vi "ErrorHandling.sendErrorEventToUI.vi"(0 "ErrorHandling in":refnum<class "ErrorHandling.lvclass">, 5 "error in (no error)":errorcluster) -> (14 "ErrorHandling out":refnum<class "ErrorHandling.lvclass">, 19 "error out":errorcluster)   [LabVIEW 2016, in "ErrorHandling.lvclass"]
doc: "Sendet das Ereignis \"errorOccurred\" an das optionale UI ErrorUI\n\n15.04.14 / sige"
uses:
  ErrorHandling.lvclass
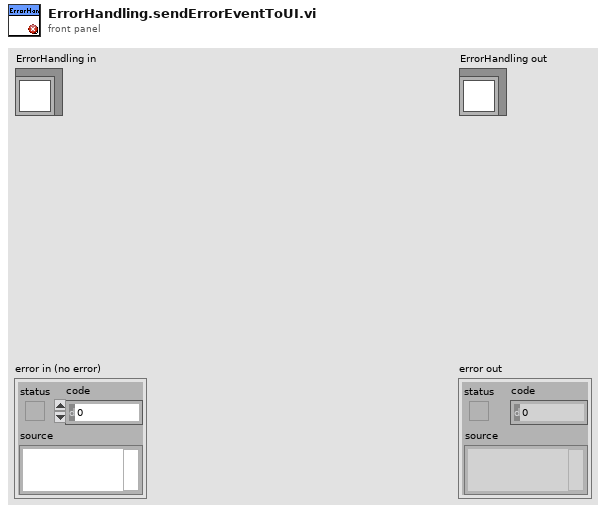
[diagram p1: front panel]
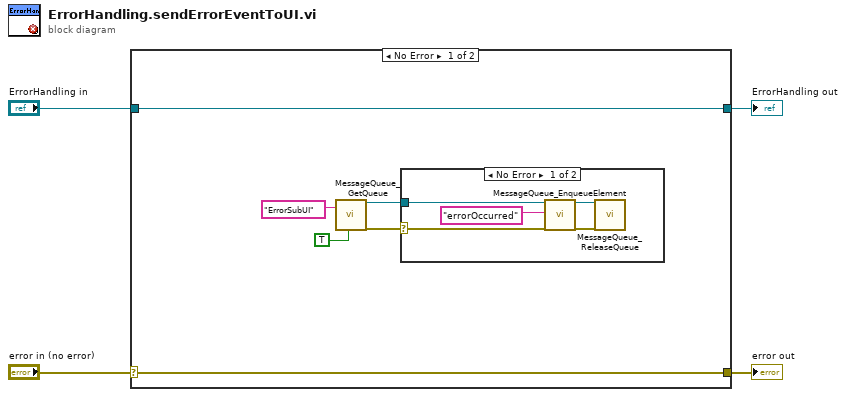
[diagram p0: block diagram]
diagram:
  n1 = case shown="No Error" "error in (no error)" {
    selector: "error in (no error)" -> [w10 w17]
    tunnel: [w10 w17] -> w3
    tunnel: [w9 w16] -> w1
    tunnel: "ErrorHandling in" -> [w9 w16]
    frame No Error {
      n2 = call "MessageQueue_GetQueue.vi"("Name"="ErrorSubUI", "CreatIfNotFount (T)"=TRUE) -> ("QueueOut"=w8:refnum<queue>, "ErrorOut"=w5:errorcluster)  [unwired: 15 in, 1 out]
      n3 = case shown="No Error" w5 {
        selector: w5 -> [w11 _]
        tunnel: w8 -> [w13 _]
        frame No Error {
          n4 = call "MessageQueue_EnqueueElement.vi"("QueueIn"=w13, "Message"="errorOccurred", "ErrorIn"=w11) -> ("QueueOut"=w14:refnum<queue>, "ErrorOut"=w12:errorcluster)  [unwired: 15 in]
          n5 = call "MessageQueue_ReleaseQueue.vi"("QueueIn"=w14, "ErrorIn"=w12) -> ()  [unwired: 15 in, 3 out]
        }
        frame Error {
        }
      }
    }
    frame Error {
    }
  }
  "error out" <- w3
  "ErrorHandling out" <- w1
